vi "TranslatorBooster Search Function Name Test.vi"(8 "error in":errorcluster, 9 "Func. prototypes file":path=path "C:/Program Files/National Instruments/LabVIEW 2014/vi.lib/Aledyne-TSXperts/Arduino Compatible Compiler for LabVIEW/addons/Complex Numbers/generated VIs/funcPrototypes.txt", 10 "Output":string[](array[string])=["out1"], 11 "Inputs":string[](array[string])=["a", "error", "b", "c"]) -> (0 "error out":errorcluster)   [LabVIEW 2014, in "Complex Numbers.lvlib"]
uses:
  <vilib>/Aledyne-TSXperts/Arduino Compatible Compiler for LabVIEW/addons/Complex Numbers/Complex Numbers.lvlib
  <vilib>/regexp/Match Regular Expression.xnode
panel:
  out "Arduino code line":string=" = (Complex*)->c_sqrt);"
  in  "Input datatypes":string[](array[string])=["adsfads", "Cluster", "fdsafadsfds", "adsffadadsf"]
  out "Line with function":string="xComplex c_sqrt()"
  out "DataType":string[](array[string])
  out "Type":string[](array[string])
  out "unsigned?":bool[](array[boolean])
  out "ref?":bool[](array[boolean])
  out "pointer?":bool[](array[boolean])
  in  "Function name":string="test1"
  out "Tokenized line":string[](array[string])=["xComplex", "c_sqrt", ""]
  out "Readed line":string="xComplex c_sqrt()"
  out "offset past match":i32=15
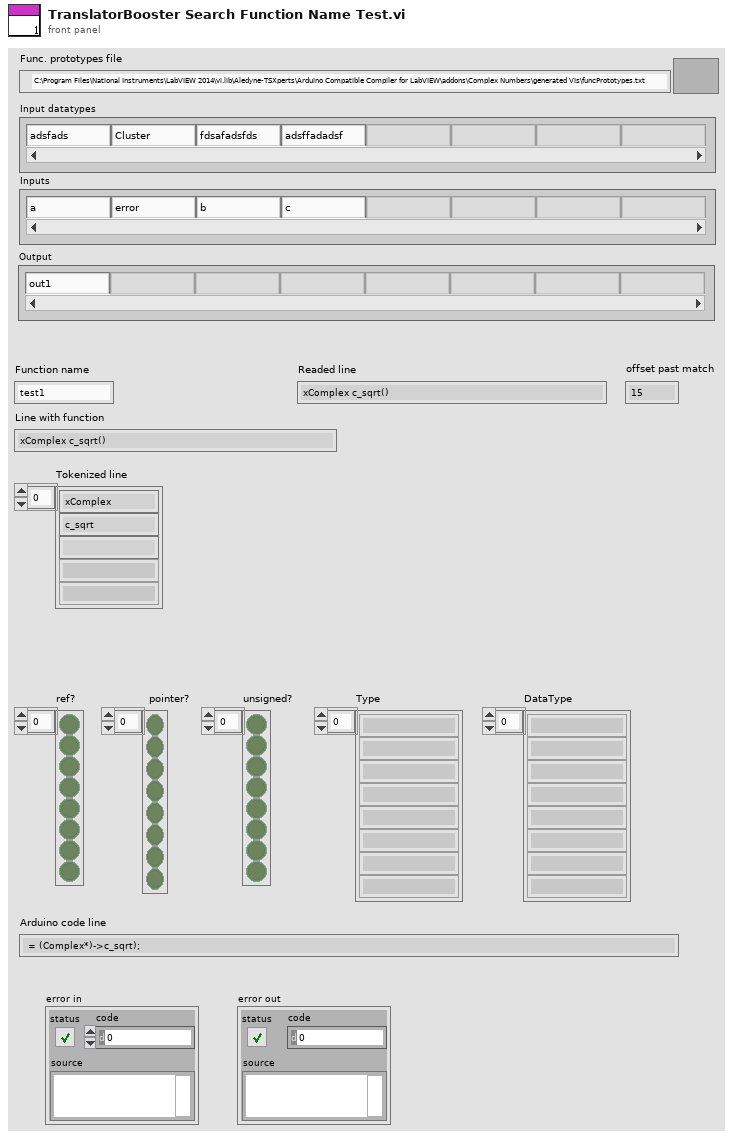
[diagram p1: front panel]
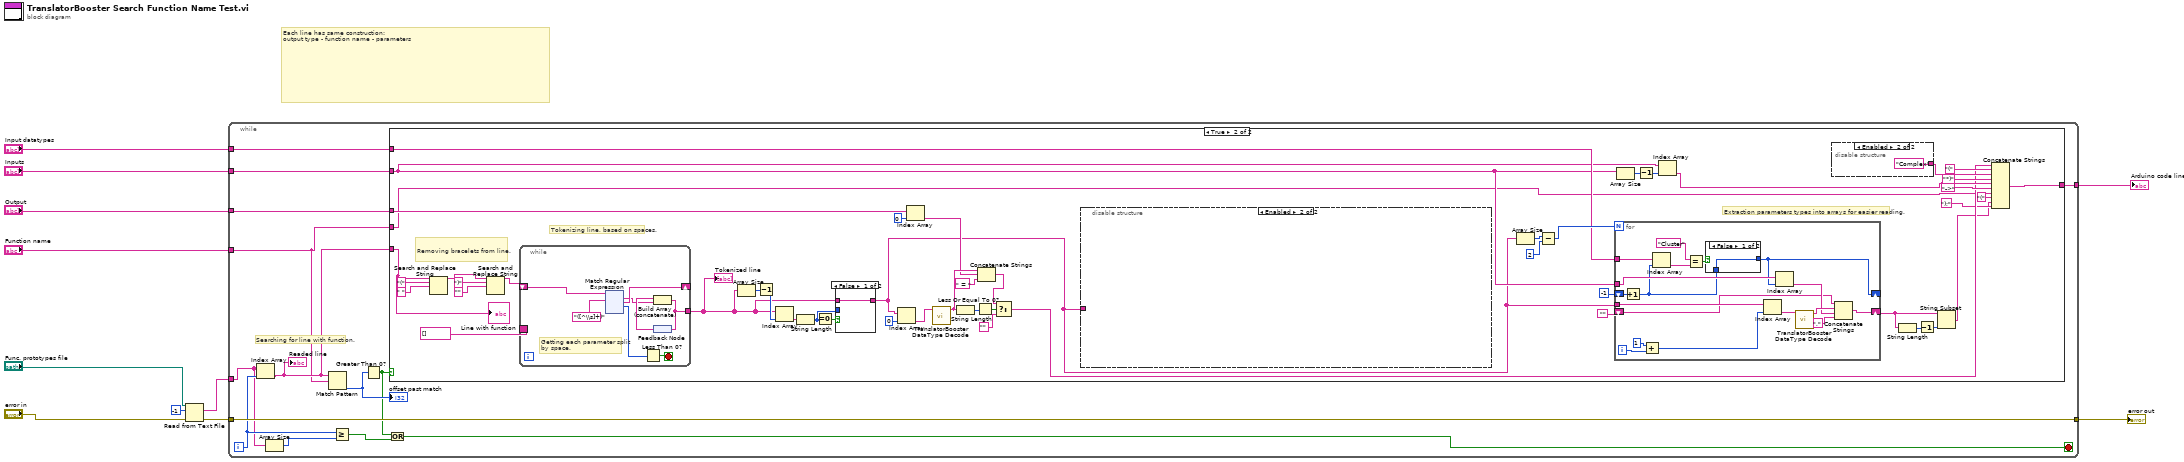
[diagram p0: block diagram]
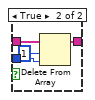
[diagram p3: hidden frame]
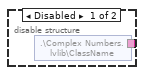
[diagram p4: hidden frame]
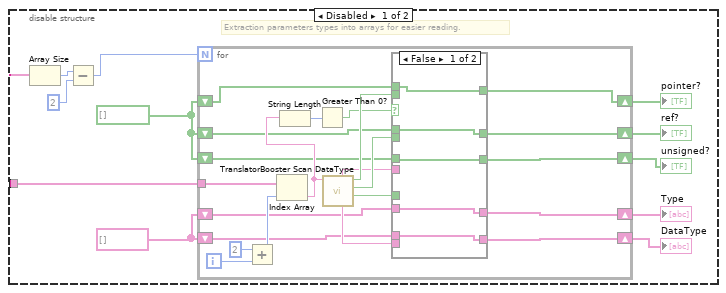
[diagram p5: hidden frame]
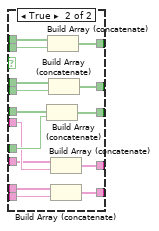
[diagram p6: hidden frame]
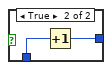
[diagram p7: hidden frame]
diagram:
  # "Each line has same construction:\noutput type - function name - parameters"
  n1 = Read from Text File(file (use dialog)="Func. prototypes file", count=-1, error in="error in") -> (text=w9:string[], error out=w7:errorcluster)  [unwired: 1 in, 2 out]
  n2 = while {
    tunnel: "Function name" -> [w12]
    tunnel: [w25] -> w5
    tunnel: w9 -> [w17]
    tunnel: w7 -> [w25]
    tunnel: "Inputs" -> [w23]
    tunnel: "Output" -> [w22]
    tunnel: "Input datatypes" -> [w21]
    tunnel: [w20] -> w1
    i -> [w18]
    stop <- w13 stop-if-true
    # "Searching for line with function."
    n3 = Index Array(array=w17, index=w18) -> (element=w19:string)
    "Readed line" <- w19
    n4 = Array Size(array=w17) -> (size(s)=w16:i32)
    n5 = Match Pattern(string=w19, regular expression=w12) -> (offset past match=w24:i32)  [unwired: 1 in, 3 out]
    "offset past match" <- w24
    n6 = Greater Or Equal?(x=w18, y=w16) -> (x >= y?=w14:bool)
    n7 = Greater Than 0?(x=w24) -> (x > 0?=w15:bool)
    n8 = Or(x=w15, y=w14) -> (x .or. y?=w13:bool)
    n9 = case shown="True" w15 {
      tunnel: w19 -> [_ w43]
      tunnel: w23 -> [_ w49]
      tunnel: w22 -> [_ w61]
      tunnel: w21 -> [_ w52]
      tunnel: [_ w38] -> w20
      tunnel: w12 -> [_ w36]
      frame False {
      }
      frame True {
        # "Extraction parameters types into arrays for easier reading."
        # "Tokenizing line, based on spaces."
        # "Removing bracelets from line."
        n10 = Search and Replace String(input string=w43, search string="(", replace string=" " ("replace string (\"\")")) -> (result string=w69:string)  [unwired: 5 in, 3 out]
        n11 = Search and Replace String(input string=w69, search string=")", replace string="" ("replace string (\"\")")) -> (result string=w68:string)  [unwired: 5 in, 3 out]
        n12 = while {
          tunnel: [w162] -> w32
          border: string[] [] -> [_]
          shift-right: [w160] -> _
          shift-left: w68 -> [w156]
          stop <- w163 stop-if-true
          # "Getting each parameter split\nby space."
          n13 = xnode "Match Regular Expression"("input string"=w156, "regular expression"="([^\\s]+)") -> ("whole match"=w157:string, "after match"=w160:string, "offset past match"=w159:i32)  [unwired: 4 in, 2 out]
          n14 = Less Than 0?(x=w159) -> (x < 0?=w163:bool)
          n15 = feedback #1() -> (w158:string[])
          n16 = Build Array (concatenate)(w158, w157) -> (w162:string[])
          n17 = feedback-in #1(w162) -> ()
        }
        "Tokenized line" <- w32
        n18 = Array Size(array=w32) -> (size(s)=w35:i32)
        n19 = Decrement(x=w35) -> (x-1=w34:i32)
        n20 = Index Array(array=w32, index=w34) -> (element=w33:string)
        n21 = String Length(string=w33) -> (length=w31:i32)
        n22 = Equal To 0?(x=w31) -> (x = 0?=w30:bool)
        n23 = case shown="False" w30 {
          tunnel: w32 -> [w75 w79]
          tunnel: w31 -> [_ w78]
          tunnel: [w75 w76] -> w29
          frame False {
          }
          frame True {
            n24 = Delete From Array(array=w79, length=1, index=w78) -> (array with subset deleted=w76:string[])  [unwired: 1 out]
          }
        }
        n25 = Index Array(array=w29, index=0) -> (element=w63:string)
        n26 = Index Array(array=w61, index=0) -> (element=w57:string)
        n27 = call <vilib>:"TranslatorBooster DataType Decode.vi"("DataType Encoded"=w63) -> ("DataType Decoded"=w58:string)  [unwired: 10 in]
        n28 = String Length(string=w58) -> (length=w60:i32)
        n29 = Less Or Equal To 0?(x=w60) -> (x <= 0?=w59:bool)
        n30 = Concatenate Strings(w58, w57, " = " ("string")) -> (w55:string)
        n31 = Select(t=w55, s=w59, f="") -> (s? t:f=w37:string)
        n32 = disable-structure shown="Enabled" {
          disable-tunnel: w29 -> [w90 _]
          frame Disabled {
            w86 = string[] []
            w87 = bool[] []
            # "Extraction parameters types into arrays for easier reading."
            n33 = Array Size(array=w90) -> (size(s)=w92:i32)
            n34 = Subtract(x=w92, y=2 ("index")) -> (x-y=w89:i32)
            n35 = for {
              N: w89 -> [_]
              tunnel: w90 -> [w114]
              shift-right: [w102] -> w88
              shift-left: w87 -> [w103]
              shift-right: [w100] -> w82
              shift-left: w87 -> [w101]
              shift-right: [w98] -> w83
              shift-left: w87 -> [w99]
              shift-right: [w96] -> w84
              shift-left: w86 -> [w97]
              shift-right: [w94] -> w85
              shift-left: w86 -> [w95]
              i -> [w113]
              n36 = Add(x=2, y=w113) -> (x+y=w107:i32)
              n37 = Index Array(array=w114, index=w107) -> (element=w104:string)
              n38 = String Length(string=w104) -> (length=w105:i32)
              n39 = Greater Than 0?(x=w105) -> (x > 0?=w93:bool)
              n40 = call <vilib>:"TranslatorBooster Scan DataType.vi"("whole match"=w104) -> ("usnigned?"=w110:bool, "ref?"=w111:bool, "pointer?"=w112:bool, "dataType"=w109:string, "type"=w108:string)  [unwired: 6 in]
              n41 = case shown="False" w93 {
                tunnel: w112 -> [_ w134]
                tunnel: w111 -> [_ w133]
                tunnel: w110 -> [_ w132]
                tunnel: w109 -> [_ w131]
                tunnel: w108 -> [_ w130]
                tunnel: w103 -> [w119 w129]
                tunnel: [w119 w128] -> w102
                tunnel: w101 -> [w118 w127]
                tunnel: [w118 w126] -> w100
                tunnel: w99 -> [w117 w125]
                tunnel: [w117 w124] -> w98
                tunnel: w97 -> [w115 w123]
                tunnel: [w115 w122] -> w96
                tunnel: w95 -> [w116 w121]
                tunnel: [w116 w120] -> w94
                frame False {
                }
                frame True {
                  n42 = Build Array (concatenate)(w125, w132) -> (w124:bool[])
                  n43 = Build Array (concatenate)(w129, w134) -> (w128:bool[])
                  n44 = Build Array (concatenate)(w127, w133) -> (w126:bool[])
                  n45 = Build Array (concatenate)(w121, w130) -> (w120:string[])
                  n46 = Build Array (concatenate)(w123, w131) -> (w122:string[])
                }
              }
            }
            "pointer?" <- w88
            "ref?" <- w82
            "unsigned?" <- w83
            "Type" <- w85
            "DataType" <- w84
          }
          frame Enabled {
          }
        }
        n47 = Array Size(array=w29) -> (size(s)=w64:i32)
        n48 = Subtract(x=w64, y=2 ("index")) -> (x-y=w66:i32)
        n49 = for {
          N: w66 -> [_]
          tunnel: w29 -> [w152]
          shift-right: [w136] -> _
          shift-left: -1 ("y") -> [w145]
          tunnel: w52 -> [w143]
          tunnel: w49 -> [w144]
          shift-right: [w139] -> w39
          shift-left: "" -> [w135]
          i -> [w148]
          n50 = Increment(x=w145) -> (x+1=w137:i32)
          n51 = Add(x=1, y=w148) -> (x+y=w151:i32)
          n52 = Index Array(array=w143, index=w137) -> (element=w142:string)
          n53 = Equal?(x="Cluster", y=w142) -> (x = y?=w140:bool)
          n54 = case shown="False" w140 {
            tunnel: w137 -> [w153 w155]
            tunnel: [w153 w154] -> w136
            frame False {
            }
            frame True {
              n55 = Increment(x=w155) -> (x+1=w154:i32)
            }
          }
          n56 = Index Array(array=w152, index=w151) -> (element=w149:string)
          n57 = Index Array(array=w144, index=w136) -> (element=w146:string)
          n58 = call <vilib>:"TranslatorBooster DataType Decode.vi"("DataType Encoded"=w149) -> ("DataType Decoded"=w147:string)  [unwired: 10 in]
          n59 = Concatenate Strings(w135, w147, w146, "," ("string")) -> (w139:string)
        }
        n60 = Array Size(array=w49) -> (size(s)=w51:i32)
        n61 = Decrement(x=w51) -> (x-1=w50:i32)
        n62 = Index Array(array=w49, index=w50) -> (element=w45:string)
        n63 = disable-structure shown="Enabled" {
          disable-tunnel: [w80 "Complex" ("String")] -> w48
          frame Disabled {
            n64 = shared-variable ".\\Complex Numbers.lvlib\\ClassName"() -> (w80:string)  [unwired: 1 in, 1 out]
          }
          frame Enabled {
          }
        }
        n65 = String Length(string=w39) -> (length=w40:i32)
        n66 = Decrement(x=w40) -> (x-1=w41:i32)
        n67 = String Subset(string=w39, length (rest)=w41) -> (substring=w27:string)  [unwired: 1 in]
        n68 = Concatenate Strings(w37, "(" ("string"), w48, "*)" ("string"), w45, "->" ("string"), w36, "(" ("string"), w27, ");" ("string")) -> (w38:string)
        "Line with function" <- w43
      }
    }
  }
  "error out" <- w5
  "Arduino code line" <- w1
